vi "Build Broadcast Msg.vi"(8 "error in (no error)":errorcluster, 10 "Brower Controller_Q":refnum<class "Message Enqueuer.lvclass">, 11 "Control Builder in":refnum<class "GUI Control Builder.lvclass">) -> (0 "error out":errorcluster, 3 "Control Builder out":refnum<class "GUI Control Builder.lvclass">)   [LabVIEW 2015, in "GUI Control Builder.lvclass"]
uses:
  GUI Control Builder.lvclass
  <vilib>/ActorFramework/Message Enqueuer/Message Enqueuer.lvclass
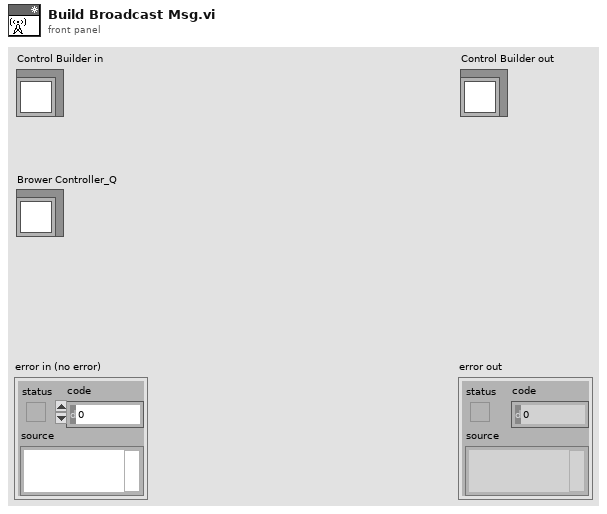
[diagram p1: front panel]
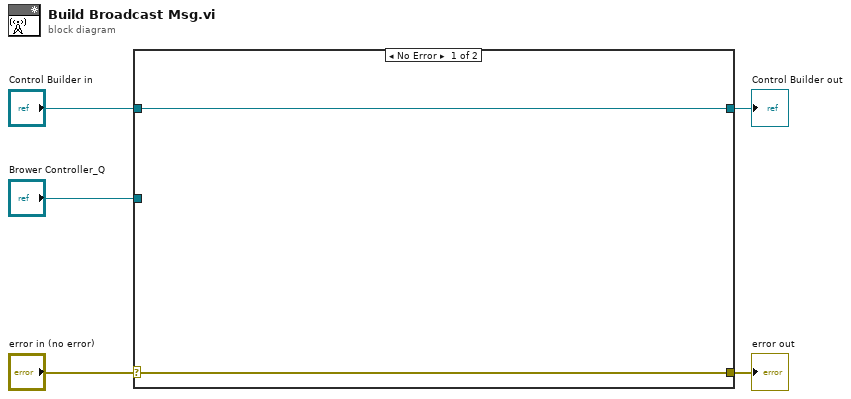
[diagram p0: block diagram]
diagram:
  n1 = case shown="No Error" "error in (no error)" {
    selector: "error in (no error)" -> [w6 w9]
    tunnel: [w6 w9] -> w4
    tunnel: [w7 w8] -> w2
    tunnel: "Control Builder in" -> [w7 w8]
    tunnel: "Brower Controller_Q" -> [_ _]
    frame No Error {
    }
    frame Error {
    }
  }
  "error out" <- w4
  "Control Builder out" <- w2
